vi "getControllerDeviceId.vi"(0 "reference (in)":refnum<class "_Controller.lvclass">, 5 "error in (no error)":errorcluster) -> (14 "reference (out)":refnum<class "_Controller.lvclass">, 16 "device_id (out)":string, 19 "error out":errorcluster)   [LabVIEW 2013, in "classes.lvlib" / "_Controller.lvclass"]
doc: "Retreive the Device ID\n\n<B>Kod Integrations, LLC</B>\n4835 Marianne Drive\nMount Airy, MD 21771\nhttp://www.kodintegrations.com\nemail: info@kodintegrations.com\nphone: (240) 687-1288"
uses:
  _Controller.lvclass
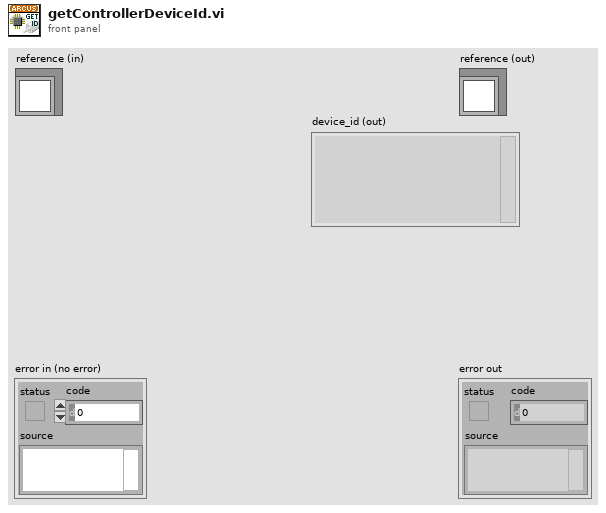
[diagram p1: front panel]
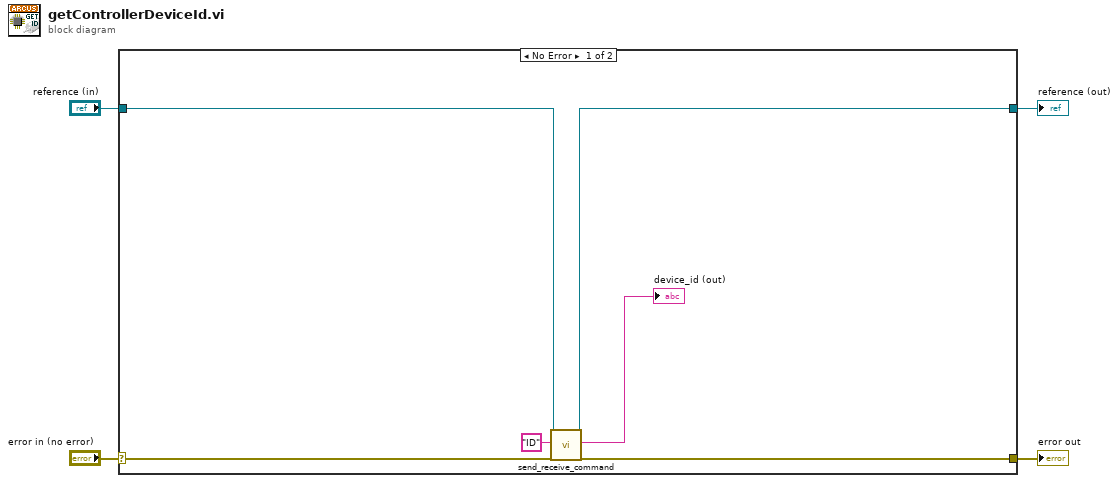
[diagram p0: block diagram]
diagram:
  n1 = case shown="No Error" "error in (no error)" {
    selector: "error in (no error)" -> [w8 w12]
    tunnel: [w7 w12] -> w3
    tunnel: [w9 w11] -> w1
    tunnel: "reference (in)" -> [w10 w11]
    frame No Error {
      n2 = call "send_receive_command.vi"("reference (in)"=w10, "ASCII Command (in)"="ID", "error in (no error)"=w8) -> ("reference (out)"=w9:refnum<class "_Controller.lvclass">, "response (out)"=→"device_id (out)":string, "error out"=w7:errorcluster)  [unwired: 12 in, 2 out]
    }
    frame Error {
    }
  }
  "error out" <- w3
  "reference (out)" <- w1
